vi "Check-Mapping-characteristics.vi"(8 "error in":errorcluster, 9 "Temp. params. ref.":refnum<data-value>, 10 "Analysis params. ref.":refnum<data-value>, 11 "Map characteristics":refnum<vi>) -> (0 "error IO":errorcluster)   [LabVIEW 2013, in "CameraVision.lvlib" / "CV-UI.lvclass"]
doc: "This function disables choices for the 'Map characteristic' front panel control depending on the chosen processing parameters."
uses:
  CV-UI.lvclass
  Main/Analysis/CV-Analysis.lvclass
  Main/Temperature/CV-Temperature.lvclass
  Main/Temperature/CV-Temperature.lvclass/CV-Temperature.ctl
  Main/Analysis/CV-Analysis.lvclass/CV-Analysis.ctl
  Main/Analysis/Read Image characteristics.vi
  Main/Analysis/Read Melt-pool characteristics.vi
  Main/Temperature/Read Temperature value.vi
  Main/Mapping/CV-Mapping.lvclass
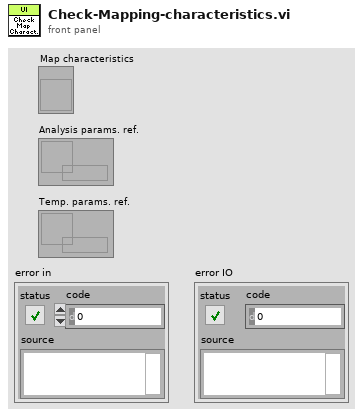
[diagram p1: front panel]
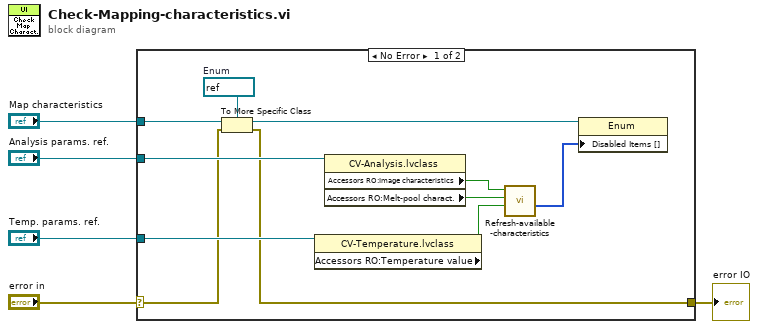
[diagram p0: block diagram]
diagram:
  n1 = case shown="No Error" "error in" {
    selector: "error in" -> [w8 w17]
    tunnel: "Map characteristics" -> [w16 _]
    tunnel: [w6 w17] -> w4
    tunnel: "Analysis params. ref." -> [w15 _]
    tunnel: "Temp. params. ref." -> [w12 _]
    frame No Error {
      w7 = refnum<vi> refnum  # Enum
      n2 = To More Specific Class(target class=w7, reference=w16, error in=w8) -> (specific class reference=w9:refnum<vi>, error out=w6:errorcluster)
      n3 = property class="CV-Temperature.lvclass"(reference=w12) -> ("Accessors RO:Temperature value"=w11:bool)  [unwired: 1 in, 2 out]
      n4 = property class="CV-Analysis.lvclass"(reference=w15) -> ("Accessors RO:Image characteristics"=w14:bool, "Accessors RO:Melt-pool charact."=w13:bool)  [unwired: 1 in, 2 out]
      n5 = call "Refresh-available-characteristics.vi"("Temperature value"=w11, "Melt-pool charact"=w13, "Image characteristics"=w14) -> ("Unavailable indices"=w10:i32[])  [unwired: 7 in, 1 out]
      n6 = property class="Enum"(reference=w9, "Disabled Items []"=w10) -> ()  [unwired: 1 in, 2 out]
    }
    frame Error {
    }
  }
  "error IO" <- w4
